vi "Shifting Enc to RPM.vi"(10 "Encoder Value":dbl, 11 "Current Gear":bool) -> (3 "RPM":dbl)   [LabVIEW 2015]
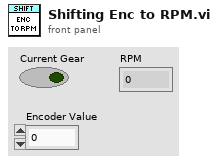
[diagram p1: front panel]
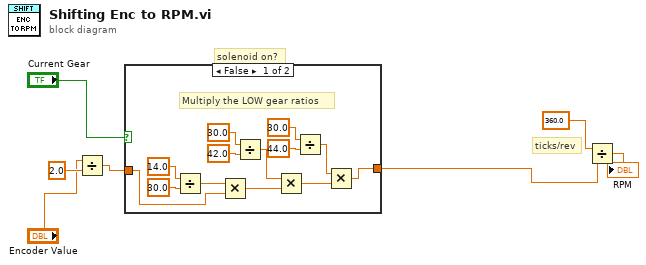
[diagram p0: block diagram]
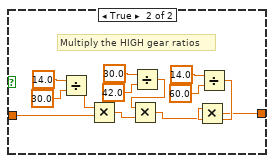
[diagram p2: hidden frame]
diagram:
  # "ticks/rev"
  # "solenoid on?"
  n1 = Divide(x="Encoder Value", y=2.0) -> (x/y=w7:dbl)
  n2 = case shown="False" "Current Gear" {
    tunnel: [w9 w22] -> w5
    tunnel: w7 -> [w8 w21]
    frame False {
      # "Multiply the LOW gear ratios"
      n3 = Divide(x=14.0, y=30.0) -> (x/y=w10:dbl)
      n4 = Multiply(x=w10, y=w8) -> (x*y=w13:dbl)
      n5 = Divide(x=30.0, y=42.0) -> (x/y=w16:dbl)
      n6 = Multiply(x=w16, y=w13) -> (x*y=w20:dbl)
      n7 = Divide(x=30.0, y=44.0) -> (x/y=w17:dbl)
      n8 = Multiply(x=w17, y=w20) -> (x*y=w9:dbl)
    }
    frame True {
      # "Multiply the HIGH gear ratios"
      n9 = Divide(x=14.0, y=30.0) -> (x/y=w33:dbl)
      n10 = Multiply(x=w33, y=w21) -> (x*y=w30:dbl)
      n11 = Divide(x=30.0, y=42.0) -> (x/y=w27:dbl)
      n12 = Multiply(x=w27, y=w30) -> (x*y=w23:dbl)
      n13 = Divide(x=14.0, y=60.0) -> (x/y=w26:dbl)
      n14 = Multiply(x=w26, y=w23) -> (x*y=w22:dbl)
    }
  }
  n15 = Divide(x=360.0, y=w5) -> (x/y=→"RPM":dbl)
